vi "Set Pin Infos.vi"(0 "Display State In":T3, 7 "Pin Info Array":T1, 9 "Container State":T4, 11 "error in (no error)":errorcluster) -> (4 "Display State Out":T3, 15 "error out":errorcluster)   [LabVIEW 2021, in "myRIO MXP.xctl"]
uses:
  <vilib>/myRIO/Common/Instrument Driver Framework/Utilities/xctls/myRIO MXP/myRIO MXP.xctl
  <vilib>/_xctls/Container State.ctl
  <vilib>/myRIO/Common/Instrument Driver Framework/Utilities/xctls/myRIO MXP/State.ctl
  <vilib>/myRIO/Common/Instrument Driver Framework/Utilities/xctls/utilities/typedefs/myRIOXC Pin Info Array.ctl
  <vilib>/myRIO/Common/Instrument Driver Framework/Utilities/xctls/utilities/typedefs/myRIOXC Pin Info.ctl
  <vilib>/myRIO/Common/Instrument Driver Framework/Utilities/xctls/utilities/vis/myRIOXC Set Pin Info.vi
  <vilib>/_xctls/XControlSupport.lvlib
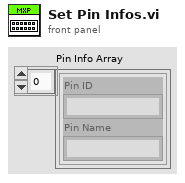
[diagram p1: front panel]
types:
  T1 = typedef "myRIOXC Pin Info Array.ctl" = T2[]
  T2 = typedef "myRIOXC Pin Info.ctl" = cluster{"Pin ID":string, "Pin Name":string}
  T3 = typedef "myRIO MXP.xctl/State.ctl" = cluster{"Pin Disabled?":enum8{"Enabled", "Disabled", "Disabled and Grayed Out"}[], "Pin Name":string[]}
  T4 = typedef "XControlSupport.lvlib/Container State.ctl" = cluster{"Indicator?":bool, "Run Mode?":bool, " Refnum":refnum<vi>}
  T5 = typedef "myRIOXC Display State.ctl" = cluster{"Pin Disabled?":enum8{"Enabled", "Disabled", "Disabled and Grayed Out"}[], "Pin Name":string[]}
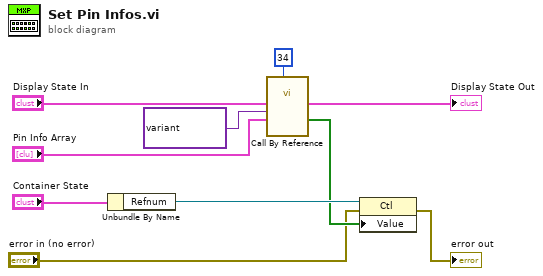
[diagram p0: block diagram]
diagram:
  n1 = Unbundle By Name("Container State") -> ("Refnum"=w6:refnum<vi>)
  n2 = call-by-ref "?"("Size"=34, "Pin Name Array"="Pin Info Array", "Pin ID Map"=variant("Pin 1"=variant(i32 0), "Pin 10"=variant(i32 9), "Pin 11"=variant(i32 10), "Pin 12"=variant(i32 11), "Pin 13"=variant(i32 12), "Pin 14"=variant(i32 13), "Pin 15"=variant(i32 14), "Pin 16"=variant(i32 15), "Pin 17"=variant(i32 16), "Pin 18"=variant(i32 17), "Pin 19"=variant(i32 18), "Pin 2"=variant(i32 1), "Pin 20"=variant(i32 19), "Pin 21"=variant(i32 20), "Pin 22"=variant(i32 21), "Pin 23"=variant(i32 22), "Pin 24"=variant(i32 23), "Pin 25"=variant(i32 24), "Pin 26"=variant(i32 25), "Pin 27"=variant(i32 26), "Pin 28"=variant(i32 27), "Pin 29"=variant(i32 28), "Pin 3"=variant(i32 2), "Pin 30"=variant(i32 29), "Pin 31"=variant(i32 30), "Pin 32"=variant(i32 31), "Pin 33"=variant(i32 32), "Pin 34"=variant(i32 33), "Pin 4"=variant(i32 3), "Pin 5"=variant(i32 4), "Pin 6"=variant(i32 5), "Pin 7"=variant(i32 6), "Pin 8"=variant(i32 7), "Pin 9"=variant(i32 8)) ("myRIO MXP"), "Display State In in"="Display State In") -> ("Data"=w5:bool[], "Display State In out"=→"Display State Out":T5)  [unwired: 8 in, 2 out]
  n3 = property class="Ctl"(reference=w6, error in="error in (no error)", "Value"=w5) -> (error out=→"error out":errorcluster)  [unwired: 1 out]
